vi "CallFacialClassFunction_IMAQ.vi"(8 "error in (no error)":errorcluster, 9 "Function or Method Name":string="findFaces", 10 "image":T1, 11 "reference in":refnum<class "ImageFacialDetection.lvclass">) -> (0 "error out":errorcluster, 2 "image with faces":T1, 3 "reference out":refnum<class "ImageFacialDetection.lvclass">)   [LabVIEW 2017, in "ImageFacialDetection.lvclass"]
doc: "uses the image classification in python with openCV to detect faces in an image using Haar Cascades"
uses:
  ImageFacialDetection.lvclass
  <vilib>/vision/Image Controls.llb/IMAQ Image.ctl
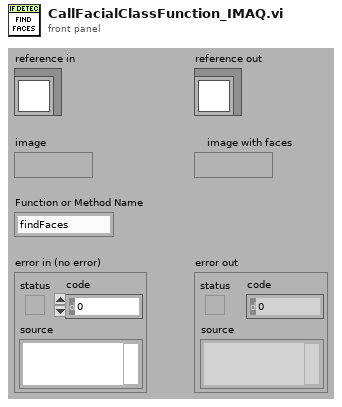
[diagram p1: front panel]
types:
  T1 = typedef "IMAQ Image.ctl" = refnum<image>
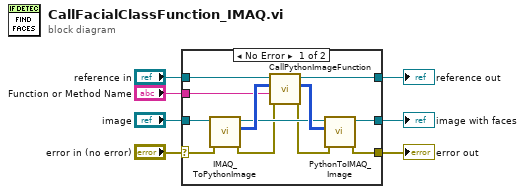
[diagram p0: block diagram]
diagram:
  n1 = case shown="No Error" "error in (no error)" {
    selector: "error in (no error)" -> [w12 w21]
    tunnel: [w9 w21] -> w6
    tunnel: [w18 w20] -> w4
    tunnel: "reference in" -> [w19 w20]
    tunnel: "image" -> [w17 _]
    tunnel: [w15 _] -> w2
    tunnel: "Function or Method Name" -> [w8 _]
    frame No Error {
      n2 = call "IMAQ_ToPythonImage.vi"("error in (no error)"=w12, "IMAQ Image in"=w17) -> ("error out"=w11:errorcluster, "Python Image Data"=w14:u8[][][], "IMAQ Image dup"=w13:T1)  [unwired: 7 in]
      n3 = call "CallPythonImageFunction.vi"("error in (no error)"=w11, "Function or Method Name"=w8, "Python Image Data in"=w14, "reference in"=w19) -> ("error out"=w10:errorcluster, "Python Image Data out"=w16:u8[][][], "reference out"=w18:refnum<class "ImageFacialDetection.lvclass">)  [unwired: 5 in]
      n4 = call "PythonToIMAQ_Image.vi"("error in (no error)"=w10, "Python Image"=w16, "IMAQ Image in"=w13) -> ("error out"=w9:errorcluster, "IMAQ Image out"=w15:T1)  [unwired: 7 in]
    }
    frame Error {
    }
  }
  "error out" <- w6
  "reference out" <- w4
  "image with faces" <- w2
